vi "GenCM-List Connected Signals.vi"(0 "Path":path, 11 "error in (no error)":errorcluster) -> (4 "Analog Outputs":string[](array[string]), 6 "Analog Inputs":string[](array[string]), 8 "Digital Outputs":string[](array[string]), 10 "Digital Inputs":string[](array[string]), 15 "error out":errorcluster)   [LabVIEW 2020]
uses:
  <vilib>/Utility/config.llb/Read Key (String).vi
  <vilib>/Utility/config.llb/NI_LVConfig.lvlib
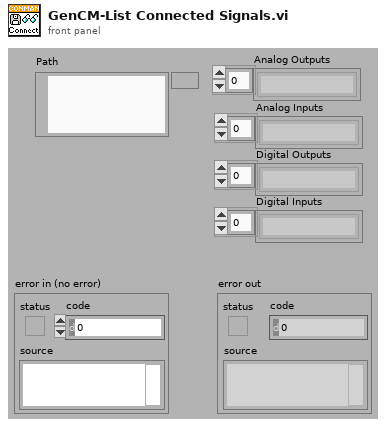
[diagram p1: front panel]
types:
  T1 = typedef "NI_LVConfig.lvlib/Config Data RefNum.ctl" = refnum<k1>
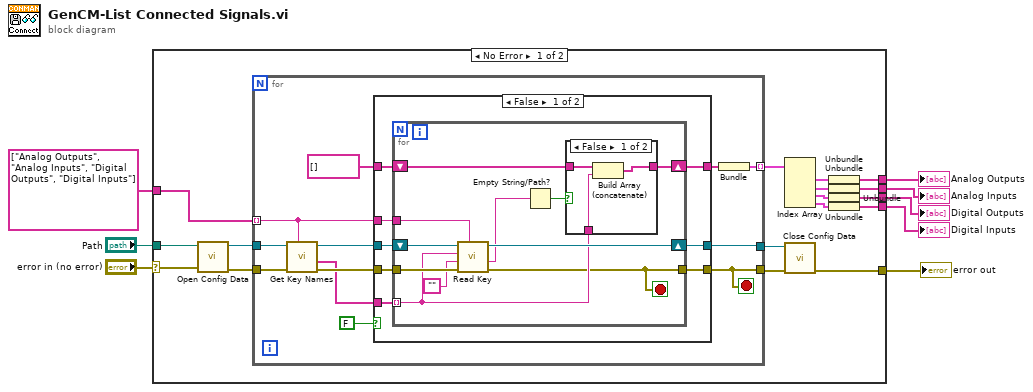
[diagram p0: block diagram]
diagram:
  n1 = case shown="No Error" "error in (no error)" {
    selector: "error in (no error)" -> [w25 w64]
    tunnel: [w24 w64] -> w7
    tunnel: "Path" -> [w23 _]
    tunnel: string[] ["Analog Outputs", "Analog Inputs", "Digital Outputs", "Digital Inputs"] -> [w22 _]
    tunnel: [w12 _] -> w4
    tunnel: [w11 _] -> w3
    tunnel: [w10 _] -> w2
    tunnel: [w9 _] -> w1
    frame No Error {
      n2 = call <vilib>:"Open Config Data.vi"("error in (no error)"=w25, "configuration file path"=w23) -> ("error out"=w18:errorcluster, "refnum"=w19:T1)  [unwired: 7 in, 1 out]
      n3 = for {
        tunnel: w19 -> [w34]
        tunnel: [w37] -> w21
        tunnel: w18 -> [w33]
        tunnel: [w26] -> w20
        tunnel: w22 -> [w30] mode=indexing
        tunnel: [w27] -> w17 mode=indexing
        stop <- w26 stop-if-true
        n4 = call <vilib>:"Get Key Names.vi"("section"=w30, "error in (no error)"=w33, "refnum"=w34) -> ("error out"=w31:errorcluster, "key names"=w29:string[], "refnum out"=w32:T1)  [unwired: 5 in, 1 out]
        n5 = case shown="False" FALSE {
          tunnel: w32 -> [w45 w62]
          tunnel: string[] [] -> [w44 w63]
          tunnel: [w43 w63] -> w36
          tunnel: [w42 w62] -> w37
          tunnel: w29 -> [w41 _]
          tunnel: w31 -> [w40 w61]
          tunnel: [w39 w61] -> w26
          tunnel: w30 -> [w38 _]
          frame False {
            n6 = for {
              tunnel: w41 -> [w49] mode=indexing
              shift-right: [w53] -> w43
              shift-left: w44 -> [w54]
              tunnel: w40 -> [w56]
              tunnel: [w47] -> w39
              tunnel: w38 -> [w48]
              shift-right: [w52] -> w42
              shift-left: w45 -> [w55]
              stop <- w47 stop-if-true
              n7 = call-poly <vilib>:"Read Key.vi"("section"=w48, "error in (no error)"=w56, "default value"="", "key"=w49, "refnum"=w55) -> ("error out"=w47:errorcluster, "value"=w50:string, "refnum out"=w52:T1)  [unwired: 3 in, 1 out]
              n8 = Empty String/Path?(string/path=w50) -> (empty?=w51:bool)
              n9 = case shown="False" w51 {
                tunnel: w54 -> [w59 w60]
                tunnel: [w58 w60] -> w53
                tunnel: w49 -> [w57 _]
                frame False {
                  n10 = Build Array (concatenate)(w59, w57) -> (w58:string[])
                }
                frame True {
                }
              }
            }
          }
          frame True {
          }
        }
        n11 = Bundle(w36) -> (w27:cluster{string[]})  [unwired: 1 in]
      }
      n12 = Index Array(array=w17) -> (element #1=w16:cluster{string[]}, element #2=w15:cluster{string[]}, element #3=w14:cluster{string[]}, element #4=w13:cluster{string[]})  [unwired: 4 in]
      n13 = call <vilib>:"Close Config Data.vi"("error in (no error)"=w20, "refnum"=w21) -> ("error out"=w24:errorcluster)  [unwired: 8 in, 1 out]
      n14 = Unbundle(w16) -> (w12:string[])
      n15 = Unbundle(w15) -> (w10:string[])
      n16 = Unbundle(w14) -> (w11:string[])
      n17 = Unbundle(w13) -> (w9:string[])
    }
    frame Error {
    }
  }
  "error out" <- w7
  "Analog Outputs" <- w4
  "Analog Inputs" <- w2
  "Digital Outputs" <- w3
  "Digital Inputs" <- w1
